vi "PreallocateArraysFFTW3.vi"(1 "Camera.lvclass":refnum<class "Camera.lvclass">, 2 "Scan.lvclass":refnum<class "Scan.lvclass">) -> (0 "FFTW3 input":T1)   [LabVIEW 2017]
uses:
  classes/Scans/Scan.lvclass
  classes/HardwareObjects/Camera/Camera.lvclass
  classes/Scans/Scan.lvclass/Scan.ctl
  classes/HardwareObjects/Camera/Camera.lvclass/Camera.ctl
  classes/HardwareObjects/Camera/Read Camera Dimensions.vi
  classes/Scans/Read Total A-scans per frame.vi
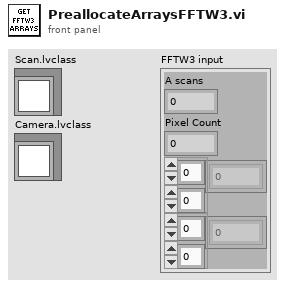
[diagram p1: front panel]
types:
  T1 = cluster{"A scans":dbl, "Pixel Count":u16, dbl[][], cdb[][]}
  T2 = cluster{"Total A-scans per frame":dbl, "Pixel Count":u16, dbl[][], cdb[][]}
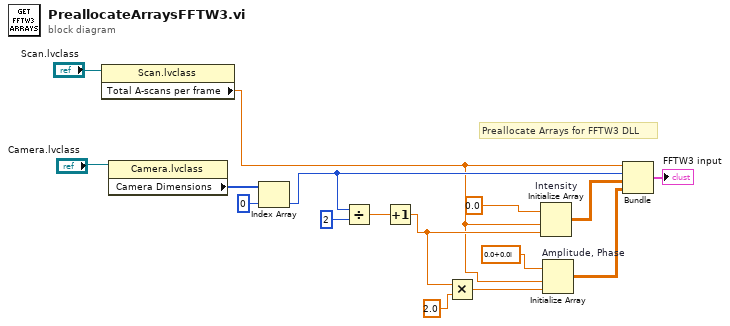
[diagram p0: block diagram]
diagram:
  # "Preallocate Arrays for FFTW3 DLL"
  n1 = property class="Scan.lvclass"(reference="Scan.lvclass") -> ("Total A-scans per frame"=w1:dbl)  [unwired: 1 in, 2 out]
  n2 = property class="Camera.lvclass"(reference="Camera.lvclass") -> ("Camera Dimensions"=w5:u16[])  [unwired: 1 in, 2 out]
  n3 = Index Array(array=w5, index=0) -> (element=w2:u16)
  n4 = Divide(x=w2, y=2) -> (x/y=w12:dbl)
  n5 = Increment(x=w12) -> (x+1=w11:dbl)
  n6 = Multiply(x=w11, y=2.0) -> (x*y=w10:dbl)
  n7 = Initialize Array "Intensity"(0.0 ("element"), w1, w11) -> (w14:dbl[][])
  n8 = Initialize Array "Amplitude, Phase"(cdb 0.0+0.0i ("element"), w1, w10) -> (w15:cdb[][])
  n9 = Bundle("Total A-scans per frame"=w1, "Pixel Count"=w2, w14, w15) -> (→"FFTW3 input":T2)  [unwired: 1 in]
